vi "Frecuencia meas.vi"(8 "error in (no error)":errorcluster, 10 "Frecuencia":dbl, 11 "Measurement GEN in":refnum<class "Measurement GEN.lvclass">) -> (0 "error out":errorcluster, 3 "Measurement GEN out":refnum<class "Measurement GEN.lvclass">)   [LabVIEW 2020, in "Measurement GEN.lvlib" / "Measurement GEN.lvclass"]
uses:
  Measurement GEN.lvclass
  Measurement GEN.lvclass/Measurement GEN.ctl
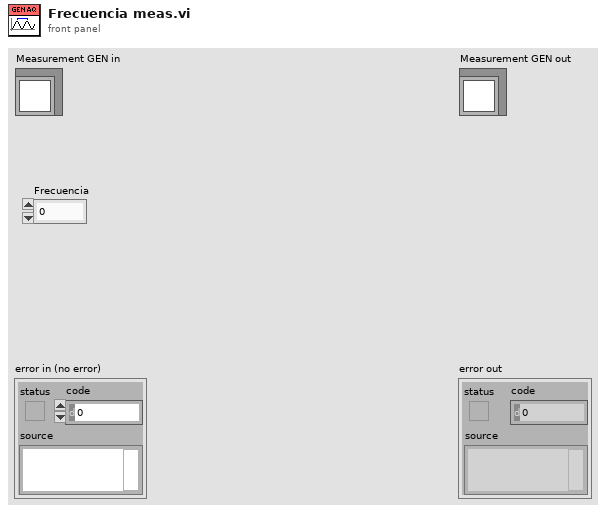
[diagram p1: front panel]
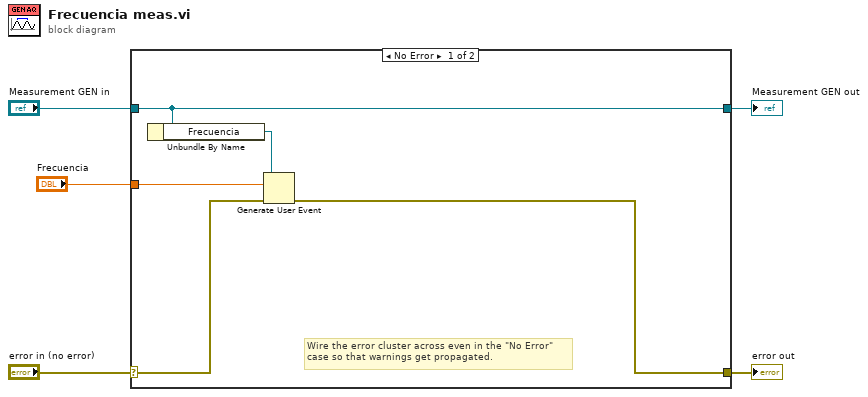
[diagram p0: block diagram]
diagram:
  n1 = case shown="No Error" "error in (no error)" {
    selector: "error in (no error)" -> [w7 w12]
    tunnel: [w6 w12] -> w4
    tunnel: [w10 w11] -> w2
    tunnel: "Measurement GEN in" -> [w10 w11]
    tunnel: "Frecuencia" -> [w8 _]
    frame No Error {
      # "Wire the error cluster across even in the \"No Error\"\ncase so that warnings get propagated."
      n2 = Unbundle By Name(w10) -> ("Frecuencia"=w9:refnum<user-event>)
      n3 = Generate User Event(user event=w9, event data cluster=w8, error in=w7) -> (error out=w6:errorcluster)  [unwired: 1 in, 1 out]
    }
    frame Error {
    }
  }
  "error out" <- w4
  "Measurement GEN out" <- w2
